vi "CreatePulseTrains.vi"() -> ()   [LabVIEW 2024]
uses:
  <vilib>/DAQmx/write.llb/DAQmx Write (Analog DBL 1Chan 1Samp).vi
  <vilib>/DAQmx/create/channels.llb/DAQmx Create Channel (AO-Voltage-Basic).vi
  <vilib>/DAQmx/miscellaneous.llb/DAQmx Fill In Error Info.vi
  <vilib>/Utility/file.llb/Write Delimited Spreadsheet (DBL).vi
panel:
  in  "Max \nRepeats":i32=100
  out "PreviousState":dbl
  out "FullStoragePath":string
  in  "physical channels":tag="NI6001/ao0"
  in  "stop":bool
  out "Waveform Graph":waveform(dbl)(graph)
  in  "Start Stimulation":bool
  in  "Time Between Stimulation (s)":dbl=5.0 min=5.0 max=200.0 step=1.0
  in  "Pulse Dur (ms)":i64=10 min=1 max=1000 step=1
  in  "Pulse Gap (ms)":i64=100 min=1 max=1000 step=1
  in  "Amp (mA)":dbl=3.0 min=0.1 max=50.0 step=0.1
  in  "Pulse Repeats":i64=3 min=1 max=1000 step=1
  out "Overview":picture
  out "Stimulation Parameters":picture
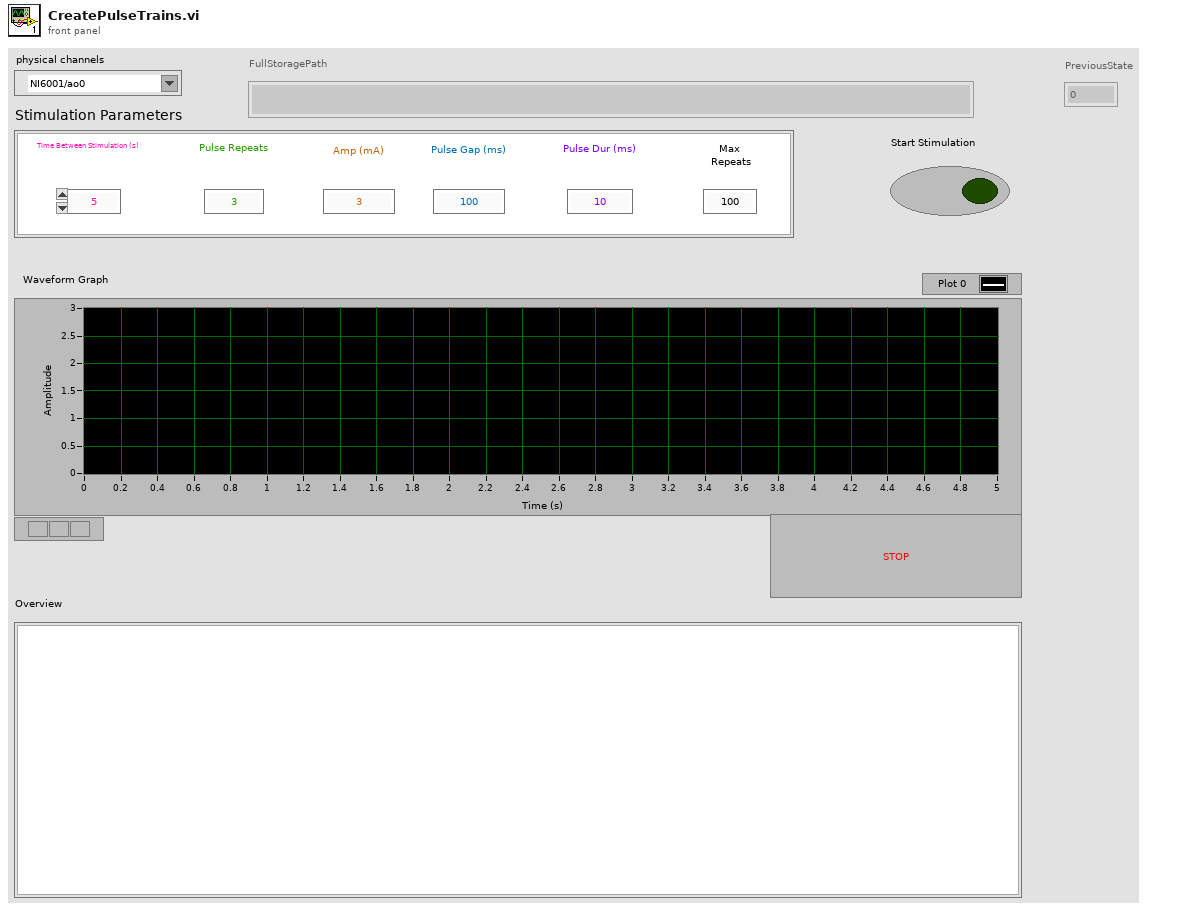
[diagram p1: front panel]
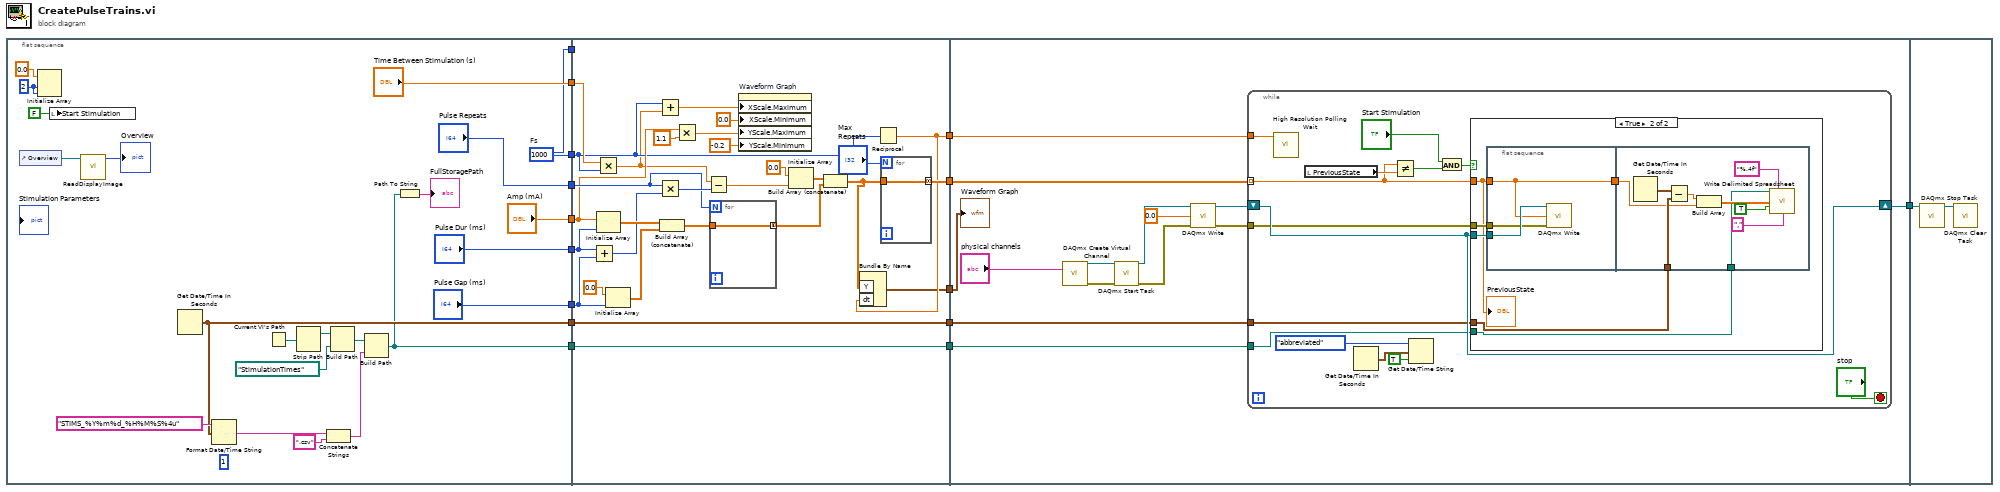
[diagram p0: block diagram]
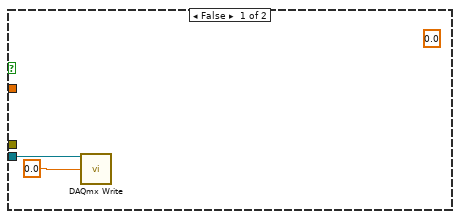
[diagram p2: hidden frame]
diagram:
  n1 = flat-sequence {
    tunnel: ["Pulse Repeats"] -> w15
    tunnel: ["Pulse Dur (ms)"] -> w14
    tunnel: ["Pulse Gap (ms)"] -> w13
    tunnel: ["Time Between Stimulation (s)"] -> w12
    tunnel: ["Amp (mA)"] -> w11
    tunnel: [w30] -> w10
    tunnel: [w30] -> w8
    tunnel: [w21] -> w4
    tunnel: [w24] -> w2
    tunnel: w15 -> [w53]
    tunnel: w14 -> [w56]
    tunnel: w13 -> [w55]
    tunnel: w12 -> [w54]
    tunnel: w11 -> [w51]
    tunnel: w10 -> [w46]
    tunnel: [w39] -> w9
    tunnel: w8 -> [_]
    tunnel: [w43] -> w7
    tunnel: [w42] -> w5
    tunnel: w4 -> [w42]
    tunnel: [w41] -> w3
    tunnel: w2 -> [w41]
    tunnel: [w38] -> w1
    tunnel: w9 -> [w77]
    tunnel: w7 -> [w79]
    tunnel: [w81] -> w6
    tunnel: w5 -> [w75]
    tunnel: w3 -> [w76]
    tunnel: w1 -> [w69]
    tunnel: w6 -> [w117]
    frame #0 {
      (unwired) 1 ("dimension size")
      w16 = 2 ("dimension size")
      w30 = 1000  # Fs
      n2 = control-ref of="Overview"() -> (w36:refnum<vi>)
      n3 = Initialize Array(0.0 ("element"), w16, w16) -> ()  [unwired: 1 out]
      n4 = local write "Start Stimulation"(FALSE ("Start Stimulation")) -> ()
      n5 = call "ReadDisplayImage.vi"("Picture in"=w36) -> ("Overview"=→"Overview":picture)  [unwired: 10 in]
      n6 = Get Date/Time In Seconds() -> (seconds since 1Jan1904=w24:timestamp)
      n7 = Format Date/Time String(time format string (%c)="STIMS_%Y%m%d_%H%M%S%4u", seconds (now)=w24) -> (date/time string=w19:string)  [unwired: 1 in]
      n8 = Current VI's Path() -> (path=w29:path)
      n9 = Strip Path(path=w29) -> (stripped path=w28:path)  [unwired: 1 out]
      n10 = Concatenate Strings(w19, ".csv" ("string")) -> (w18:string)
      n11 = Build Path(base path=w28, name or relative path=path "StimulationTimes") -> (appended path=w22:path)
      n12 = Build Path(base path=w22, name or relative path=w18) -> (appended path=w21:path)
      n13 = Path To String(path=w21) -> (string=→"FullStoragePath":string)
    }
    frame #1 {
      n14 = Add(x=w56, y=w55) -> (x+y=w59:i64)
      n15 = Multiply(x=w54, y=w46) -> (x*y=w45:dbl)
      n16 = Initialize Array(w51, w56) -> (w61:dbl[])
      n17 = Initialize Array(0.0 ("element"), w55) -> (w62:dbl[])
      n18 = Add(x=w46, y=w45) -> (x+y=w50:dbl)
      n19 = Multiply(x=w53, y=w59) -> (x*y=w60:i64)
      n20 = Build Array (concatenate)(w61, w62) -> (w66:dbl[])
      n21 = Multiply(x=w51, y=1.1) -> (x*y=w48:dbl)
      n22 = Subtract(x=w45, y=w60) -> (x-y=w63:dbl)
      n23 = for {
        N: w53 -> [_]
        tunnel: w66 -> [w68]
        tunnel: [w68] -> w65 mode=concatenating
      }
      n24 = property on="Waveform Graph" class="WFGraph (strict)"("XScale.Maximum"=w50, "XScale.Minimum"=0.0, "YScale.Maximum"=w48, "YScale.Minimum"=-0.2 ("Y Scale.Range:Minimum")) -> ()  [unwired: 2 in, 2 out]
      n25 = Initialize Array(0.0, w63) -> (w64:dbl[])
      n26 = Build Array (concatenate)(w64, w65) -> (w40:dbl[])
      n27 = Reciprocal(x=w46) -> (1/x=w39:dbl)
      n28 = Bundle By Name("Y"=w40, "dt"=w39) -> (w38:waveform(dbl))  [unwired: 1 in]
      n29 = for {
        N: "Max \nRepeats" -> [_]
        tunnel: w40 -> [w67]
        tunnel: [w67] -> w43 mode=concatenating
      }
    }
    frame #2 {
      n30 = call-poly <vilib>:"DAQmx Create Virtual Channel.vi"("physical channels"="physical channels") -> ("task out"=w82:refnum<k21>, "error out"=w78:errorcluster)  [unwired: 13 in]
      n31 = call <vilib>:"DAQmx Start Task.vi"("task/channels in"=w82, "error in"=w78) -> ("task out"=w74:refnum<k21>, "error out"=w70:errorcluster)  [unwired: 12 in]
      n32 = call-poly <vilib>:"DAQmx Write.vi"("task/channels in"=w74, "data"=0.0, "error in"=w70) -> ("task out"=w72:refnum<k21>, "error out"=w71:errorcluster)  [unwired: 10 in, 1 out]
      n33 = while {
        shift-right: [w95] -> w81
        shift-left: w72 -> [w95]
        tunnel: w79 -> [w87] mode=indexing
        tunnel: w71 -> [w94]
        tunnel: w77 -> [w93]
        tunnel: w76 -> [w89]
        tunnel: w75 -> [w83]
        stop <- "stop" stop-if-true
        n34 = call <vilib>:"High Resolution Polling Wait.vi"("seconds to wait"=w93) -> ()  [unwired: 10 in, 1 out]
        n35 = local read "PreviousState"() -> (w88:dbl)
        n36 = Get Date/Time In Seconds() -> (seconds since 1Jan1904=w92:timestamp)
        n37 = Not Equal?(x=w87, y=w88) -> (x != y?=w86:bool)
        n38 = Get Date/Time String(date format (0)=enum16{"short", "long", "abbreviated"}."abbreviated", seconds (now)=w92, want seconds? (F)=TRUE) -> ()  [unwired: 2 out]
        n39 = And(x="Start Stimulation", y=w86) -> (x .and. y?=w84:bool)
        n40 = case shown="True" w84 {
          tunnel: w95 -> [w98 w104]
          tunnel: w87 -> [_ w101]
          tunnel: w94 -> [_ w103]
          tunnel: w89 -> [_ w102]
          tunnel: w83 -> [_ w99]
          frame False {
            (unwired) 0.0 ("element")
            n41 = call-poly <vilib>:"DAQmx Write.vi"("task/channels in"=w98, "data"=0.0) -> ()  [unwired: 11 in, 3 out]
          }
          frame True {
            n42 = flat-sequence {
              tunnel: w104 -> [w107]
              tunnel: w101 -> [w105]
              tunnel: w103 -> [w106]
              tunnel: [w105] -> w100
              tunnel: w102 -> [w115]
              tunnel: w100 -> [w113]
              tunnel: w99 -> [w108]
              frame #0 {
                n43 = call-poly <vilib>:"DAQmx Write.vi"("task/channels in"=w107, "data"=w105, "error in"=w106) -> ()  [unwired: 10 in, 3 out]
              }
              frame #1 {
                n44 = Get Date/Time In Seconds() -> (seconds since 1Jan1904=w116:timestamp)
                n45 = Subtract(x=w116, y=w115) -> (x-y=w114:dbl)
                n46 = Build Array(w114, w113) -> (w109:dbl[])
                n47 = call-poly <vilib>:"Write Delimited Spreadsheet.vi"("file path (dialog if empty)"=w108, "format (%.3f)"="%.4f", "1D data"=w109, "append to file? (new file:F)"=TRUE, "delimiter (\\t)"="," ("delimiter (\\t)")) -> ()  [unwired: 9 in, 2 out]
              }
            }
            "PreviousState" <- w101
          }
        }
      }
      "Waveform Graph" <- w69
    }
    frame #3 {
      n48 = call <vilib>:"DAQmx Stop Task.vi"("task/channels in"=w117) -> ("task out"=w118:refnum<k21>)  [unwired: 13 in, 1 out]
      n49 = call <vilib>:"DAQmx Clear Task.vi"("task in"=w118) -> ()  [unwired: 14 in, 1 out]
    }
  }
